vi "DSF.Engine.Framework.Process Transfer Groups.Rx.vi"(8 "error in (no error)":errorcluster, 9 "Transfer Group indicies":i32[](array[numeric]), 10 "Plugin index":i32, 11 "Framework in":refnum<class "Framework.lvclass">) -> (0 "error out":errorcluster, 3 "Framework out":refnum<class "Framework.lvclass">)   [LabVIEW 2016, in "DSF.Engine.lvlib" / "Framework.lvclass"]
uses:
  Framework.lvclass
  Plugin/Plugin.lvclass
  Interface/DSF.Engine.Interface.Plugin.lvclass
  Interface/DSF.Engine.Interface.Plugin.Write.Command.vi
  Interface/DSF.Engine.Interface.Plugin.Read.Response.vi
  BuilderManager/DSF.Engine.BuilderManager.lvclass
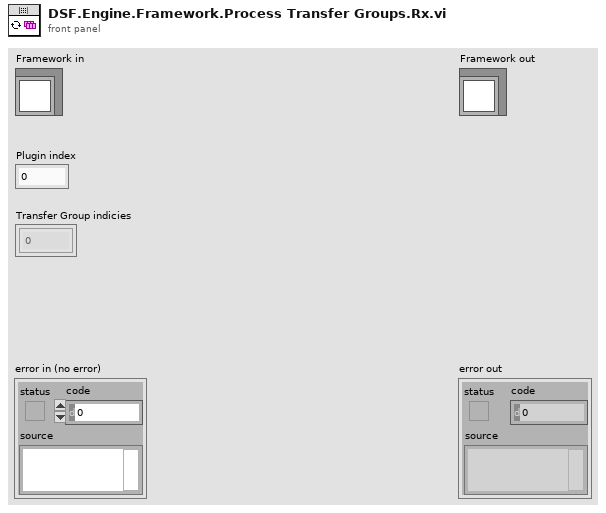
[diagram p1: front panel]
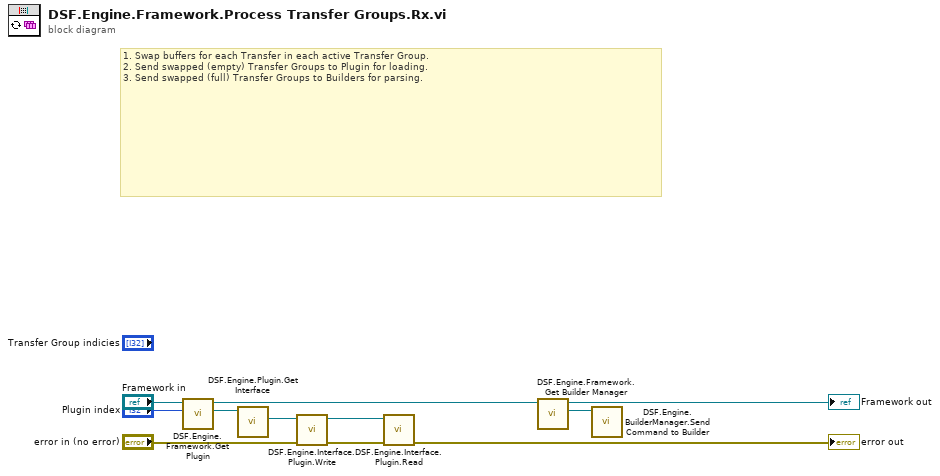
[diagram p0: block diagram]
diagram:
  # "1. Swap buffers for each Transfer in each active Transfer Group.\n2. Send swapped (empty) Transfer Groups to Plugin for loading.\n3. Send swapped (full) Transfer Groups to Builders for parsing."
  n1 = call "DSF.Engine.Framework.Get Plugin.vi"("index"="Plugin index", "Framework in"="Framework in") -> ("Plugin"=w9:refnum<class "Plugin.lvclass">, "Framework out"=w2:refnum<class "Framework.lvclass">)  [unwired: 8 in]
  n2 = call "DSF.Engine.Plugin.Get Interface.vi"("Plugin in"=w9) -> ("Interface"=w8:refnum<class "DSF.Engine.Interface.Plugin.lvclass">)  [unwired: 9 in, 1 out]
  n3 = call-poly "DSF.Engine.Interface.Plugin.Write.vi"("error in (no error)"="error in (no error)", "Plugin Interface in"=w8) -> ("error out"=w5:errorcluster, "Plugin Interface out"=w7:refnum<class "DSF.Engine.Interface.Plugin.lvclass">)  [unwired: 7 in, 1 out]
  n4 = call-poly "DSF.Engine.Interface.Plugin.Read.vi"("error in (no error)"=w5, "Plugin Interface in"=w7) -> ("error out"=→"error out":errorcluster)  [unwired: 5 in, 4 out]
  n5 = call "DSF.Engine.Framework.Get Builder Manager.vi"("Framework in"=w2) -> ("Builder Manager"=w1:refnum<class "DSF.Engine.BuilderManager.lvclass">, "Framework out"=→"Framework out":refnum<class "Framework.lvclass">)  [unwired: 9 in]
  n6 = call "DSF.Engine.BuilderManager.Send Command to Builder.vi"("Builder Manager in"=w1) -> ()  [unwired: 7 in, 4 out]
